vi "Status Clear Status.vi"(0 "VISA resource name":refnum<visa-resource-name>, 11 "error in (no error)":errorcluster) -> (4 "VISA resource name out":refnum<visa-resource-name>, 15 "error out":errorcluster)   [LabVIEW 2015, in "Chroma ATE 6310.lvlib"]
doc: "This VI executes the following actions:\n\n1. Clear these registers:\n Channel Stautus Event Register for all channels\n Channel Summary Event Register\n Questionable Status Event Register\n Standard Event Status Event Register\n\n2. Clear the Error queue\n\n3. If \"Clear Status Command\" immediately follows a program message terminator, the \"Output Queue\" and the MAV bit are also cleared."
uses:
  <instrlib>/Chroma ATE 6310/Chroma ATE 6310.lvlib
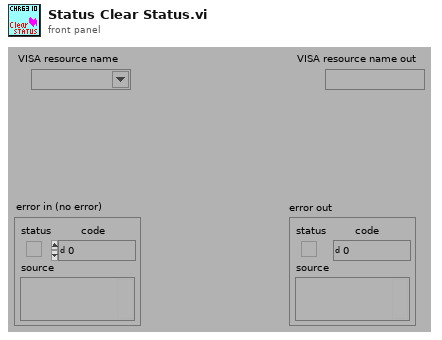
[diagram p1: front panel]
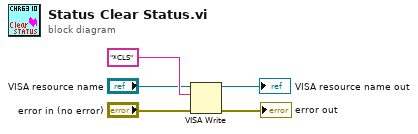
[diagram p0: block diagram]
diagram:
  n1 = VISA Write(VISA resource name="VISA resource name", write buffer="*CLS", error in (no error)="error in (no error)") -> (VISA resource name out=→"VISA resource name out":refnum<visa-resource-name>, error out=→"error out":errorcluster)  [unwired: 1 out]
